vi "Restore Startup Configuration.vi"(8 "error in (no error)":errorcluster, 10 "Startup Configuration File":path=path "C:/Data/Config/start-up.cfg", 11 "Monitor-Pulse in":refnum<class "LabActor.lvclass">) -> (0 "error out":errorcluster, 3 "Monitor-Pulse out":refnum<class "LabActor.lvclass">)   [LabVIEW 2024, in "LabActor.lvclass"]
uses:
  LabActor.lvclass
  LabActor.lvclass/LabActor.ctl
  <vilib>/Utility/error.llb/Error Cluster From Error Code.vi
  <vilib>/ErrorRing/Error Ring.xnode
  Controllers/Application Controller/Application Controller.lvclass
  <vilib>/Utility/config.llb/NI_LVConfig.lvlib
  <userlib>/_OpenG.lib/variantconfig/variantconfig.llb/openg_variant_configuration_file.lvlib
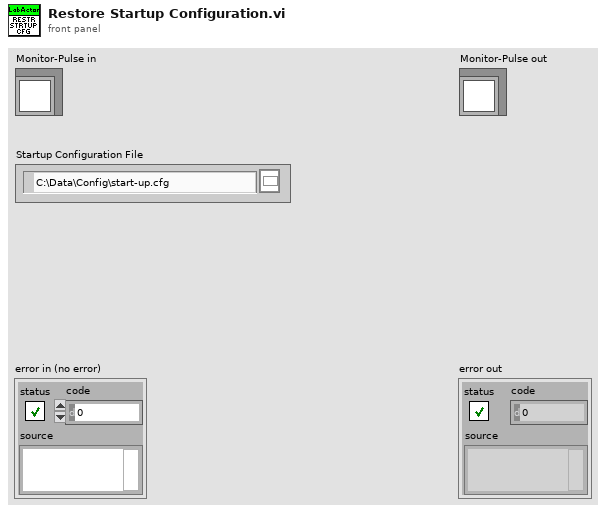
[diagram p1: front panel]
types:
  T1 = typedef "NI_LVConfig.lvlib/Config Data RefNum.ctl" = refnum<k1>
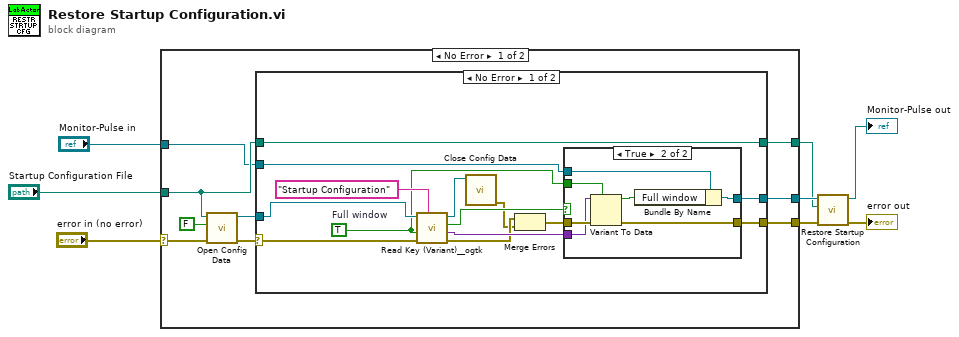
[diagram p0: block diagram]
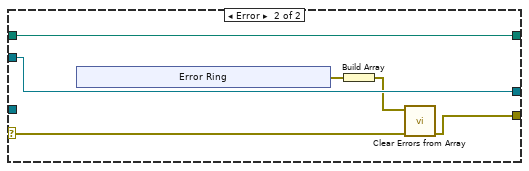
[diagram p3: hidden frame]
diagram:
  n1 = case shown="No Error" "error in (no error)" {
    selector: "error in (no error)" -> [w12 w53]
    tunnel: [w10 w53] -> w2
    tunnel: [w16 w52] -> w3
    tunnel: "Monitor-Pulse in" -> [w11 w52]
    tunnel: "Startup Configuration File" -> [w13 w51]
    tunnel: [w9 w51] -> w1
    frame No Error {
      n2 = call <vilib>:"Open Config Data.vi"("error in (no error)"=w12, "create file if necessary (T)"=FALSE, "configuration file path"=w13) -> ("error out"=w15:errorcluster, "refnum"=w17:T1)  [unwired: 6 in, 1 out]
      n3 = case shown="No Error" w15 {
        selector: w15 -> [w21 w46]
        tunnel: w11 -> [w20 w45]
        tunnel: w17 -> [w30 _]
        tunnel: [w29 w45] -> w16
        tunnel: [w27 w44] -> w10
        tunnel: w13 -> [w19 w41]
        tunnel: [w19 w41] -> w9
        frame No Error {
          w18 = TRUE  # Full window
          n4 = call <userlib>:"Read Key (Variant)__ogtk.vi"("section"="Startup Configuration", "error in (no error)"=w21, "type"=w18, "refnum"=w30) -> ("error out"=w25:errorcluster, "key-value"=w28:variant, "found?"=w26:bool, "refnum out"=w24:T1)  [unwired: 4 in]
          n5 = call <vilib>:"Close Config Data.vi"("refnum"=w24) -> ("error out"=w23:errorcluster)  [unwired: 9 in, 1 out]
          n6 = Merge Errors(w25, w23) -> (w22:errorcluster)
          n7 = case shown="True" w26 {
            tunnel: w20 -> [w33 w40]
            tunnel: [w33 w39] -> w29
            tunnel: w22 -> [w32 w38]
            tunnel: w28 -> [_ w37]
            tunnel: w18 -> [_ w36]
            tunnel: [w32 w34] -> w27
            frame False {
            }
            frame True {
              n8 = Variant To Data(error in=w38, type=w36, Variant=w37) -> (data=w35:bool, error out=w34:errorcluster)
              n9 = Bundle By Name(cluster=w40, "Full window"=w35) -> (w39:refnum<class "LabActor.lvclass">)
            }
          }
        }
        frame Error {
          n10 = xnode "Error Ring"() -> ("error out"=w43:errorcluster)
          n11 = Build Array(w43) -> (w42:errorcluster[])
          n12 = call "Clear Errors from Array.vi"("Error In"=w46, "Errors to clear"=w42) -> ("Error Out"=w44:errorcluster)  [unwired: 8 in, 1 out]
        }
      }
    }
    frame Error {
    }
  }
  n13 = call-parent "Restore Startup Configuration.vi"("error in (no error)"=w2, "Startup Configuration File"=w1, "Application Controller in"=w3) -> ("error out"=→"error out":errorcluster, "Application Controller out"=→"Monitor-Pulse out":refnum<class "LabActor.lvclass">)  [unwired: 7 in]
